vi "Create Channel Terminal.vi"(7 "Can be Indicator?":bool, 8 "error in (no error)":errorcluster, 9 "Type Descriptor":T1, 11 "VI in":refnum<vi>) -> (0 "error out":errorcluster, 2 "Ctl Refnum":refnum<vi>)   [LabVIEW 2020, in "FlexBlocks.lvlib"]
uses:
  FlexBlocks.lvlib
  Type Descriptor.ctl
  Terminal Direction.ctl
  Value Mode.ctl
  Special Terminal.ctl
  <vilib>/Utility/miscctls.llb/LVPointTypeDef.ctl
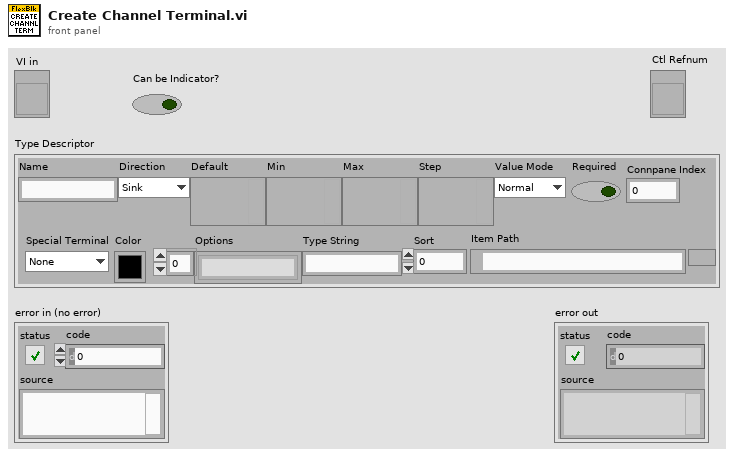
[diagram p1: front panel]
types:
  T1 = typedef "FlexBlocks.lvlib/Type Descriptor.ctl" = cluster{"Name":string, "Direction":T2, "Default":variant, "Min":variant, "Max":variant, "Step":variant, "Value Mode":T3, "Required":bool, "Connpane Index":i32, "Special Terminal":T4, "Color":u32, "Options":string[], "Type String":string, "Sort":i32, "Item Path":path}
  T2 = typedef "FlexBlocks.lvlib/Terminal Direction.ctl" = enum16{"Sink", "Source"}
  T3 = typedef "FlexBlocks.lvlib/Value Mode.ctl" = enum16{"Normal", "Range", "Select"}
  T4 = typedef "FlexBlocks.lvlib/Special Terminal.ctl" = enum16{"None", "Action", "Init", "Tag", "State in", "State out", "Error"}
  T5 = typedef "LVPointTypeDef.ctl" = cluster{"Horizontal":i16, "Vertical":i16}
  T6 = enum8{"Probe", "Diagram", "Panel Control", "3D Panel Control", "Dialog Panel Control", "Panel Indicator", "3D Panel Indicator", "Dialog Panel Indicator", "Power PC Control", "Power PC Indicator", "Silver Control", "Silver Indicator", "NXG Style Control", "NXG Style Indicator"}
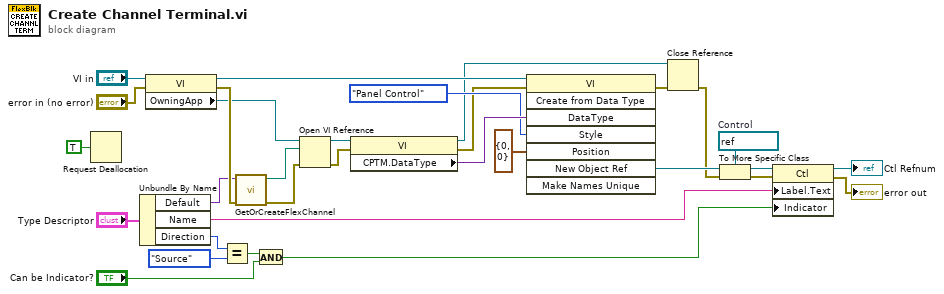
[diagram p0: block diagram]
diagram:
  w12 = refnum<vi> refnum  # Control
  n1 = Request Deallocation(TRUE ("flag")) -> ()
  n2 = Unbundle By Name("Type Descriptor") -> ("Default"=w29:variant, "Name"=w4:string, "Direction"=w28:T2)
  n3 = property class="VI"(reference="VI in", error in="error in (no error)") -> (reference out=w18:refnum<vi>, error out=w31:errorcluster, "OwningApp"=w23:refnum<vi>)
  n4 = Equal?(x=w28, y=Terminal_Direction."Source") -> (x = y?=w26:bool)
  n5 = call "GetOrCreateFlexChannel.vi"("error in (no error)"=w31, "Element Type"=w29) -> ("error out"=w1:errorcluster, "Channel Path"=w22:path)  [unwired: 8 in]
  n6 = And(x=w26, y="Can be Indicator?") -> (x .and. y?=w3:bool)
  n7 = Open VI Reference(application reference (local)=w23, vi path=w22, error in (no error)=w1) -> (vi reference=w20:refnum<vi>, error out=w19:errorcluster)  [unwired: 3 in]
  n8 = property class="VI"(reference=w20, error in=w19) -> (reference out=w9:refnum<vi>, error out=w11:errorcluster, "CPTM.DataType"=w17:variant)
  n9 = invoke class="VI" method="Create from Data Type"(reference=w18, error in=w11, "DataType"=w17, "Style"=T6."Panel Control", "Position"=T5 {"Horizontal"=0, "Vertical"=0}) -> (error out=w10:errorcluster, "New Object Ref"=w14:refnum<vi>)  [unwired: 3 in, 6 out]
  n10 = Close Reference(reference=w9, error in (no error)=w10) -> (error out=w8:errorcluster)
  n11 = To More Specific Class(target class=w12, reference=w14, error in=w8) -> (specific class reference=w13:refnum<vi>, error out=w7:errorcluster)
  n12 = property class="Ctl"(reference=w13, error in=w7, "Label.Text"=w4, "Indicator"=w3) -> (reference out=→"Ctl Refnum":refnum<vi>, error out=→"error out":errorcluster)
